vi "Lidar Functional Global.vi"(2 "Lidar Angle Data In (Degrees)":dbl[](array[numeric]), 3 "Lidar Magnitude Data In (mm)":dbl[](array[numeric]), 4 "Lidar Action":enum16{"Set Lidar Data", "Read Lidar Data"}(ring)) -> (0 "Lidar Angle Data Out (Degrees)":dbl[](array[numeric]), 1 "Lidar Magnitude Data Out (mm)":dbl[](array[numeric]))   [LabVIEW 2010]
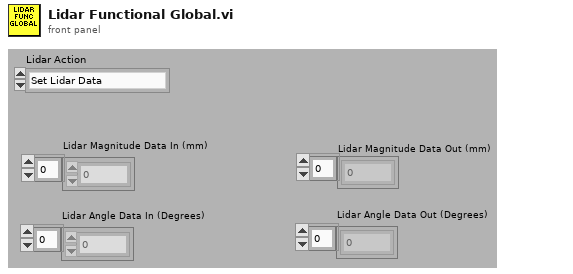
[diagram p1: front panel]
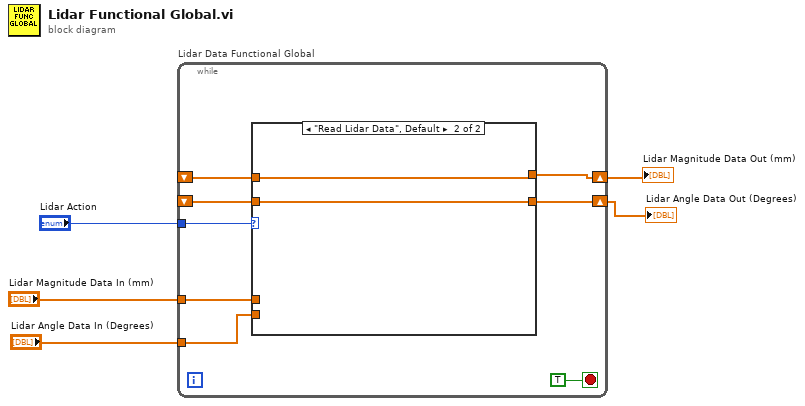
[diagram p0: block diagram]
diagram:
  n1 = while "Lidar Data Functional Global" {
    shift-right: [w10] -> w2
    shift-left: _ -> [w8]
    tunnel: "Lidar Action" -> [w13]
    shift-right: [w12] -> w1
    shift-left: _ -> [w7]
    tunnel: "Lidar Angle Data In (Degrees)" -> [w11]
    tunnel: "Lidar Magnitude Data In (mm)" -> [w9]
    stop <- TRUE stop-if-true
    n2 = case shown="\"Read Lidar Data\", Default" w13 {
      tunnel: [w15 w16] -> w12
      tunnel: w11 -> [w15 _]
      tunnel: [w14 w17] -> w10
      tunnel: w9 -> [w14 _]
      tunnel: w8 -> [_ w17]
      tunnel: w7 -> [_ w16]
      frame "Set Lidar Data" {
      }
      frame "Read Lidar Data", Default {
      }
    }
  }
  "Lidar Angle Data Out (Degrees)" <- w1
  "Lidar Magnitude Data Out (mm)" <- w2
